vi "Read Measurement (Statistics).vi"(0 "VISA resource name":refnum<visa-resource-name>, 5 "Statistics Type (0: All)":i32(ring) items=["All", "Current", "Minimum", "Maximum", "Mean", "Std Dev", "Count"], 11 "error in (no error)":errorcluster) -> (2 "Measurement Data":string[](array[string]), 3 "Current Data":dbl[](array[numeric]), 4 "VISA resource name out":refnum<visa-resource-name>, 6 "Mean Data":dbl[](array[numeric]), 8 "Minimum Data":dbl[](array[numeric]), 10 "Maximum Data":dbl[](array[numeric]), 13 "Count Data":dbl[](array[numeric]), 14 "Std Dev Data":dbl[](array[numeric]), 15 "error out":errorcluster)   [LabVIEW 2015, in "Agilent 2000 3000 X-Series.lvlib"]
doc: "Returns the measurement of static acquisition."
uses:
  <instrlib>/Agilent 2000 3000 X-Series/Agilent 2000 3000 X-Series.lvlib
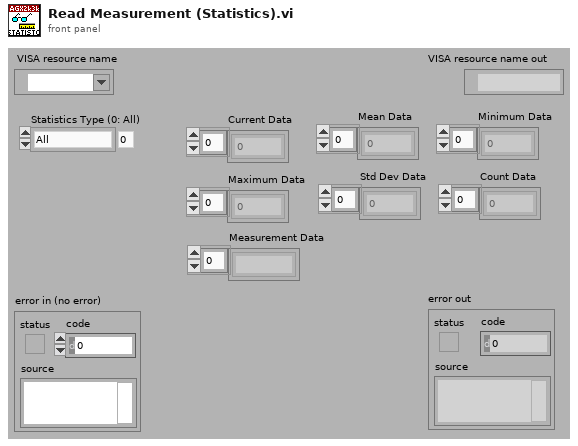
[diagram p1: front panel]
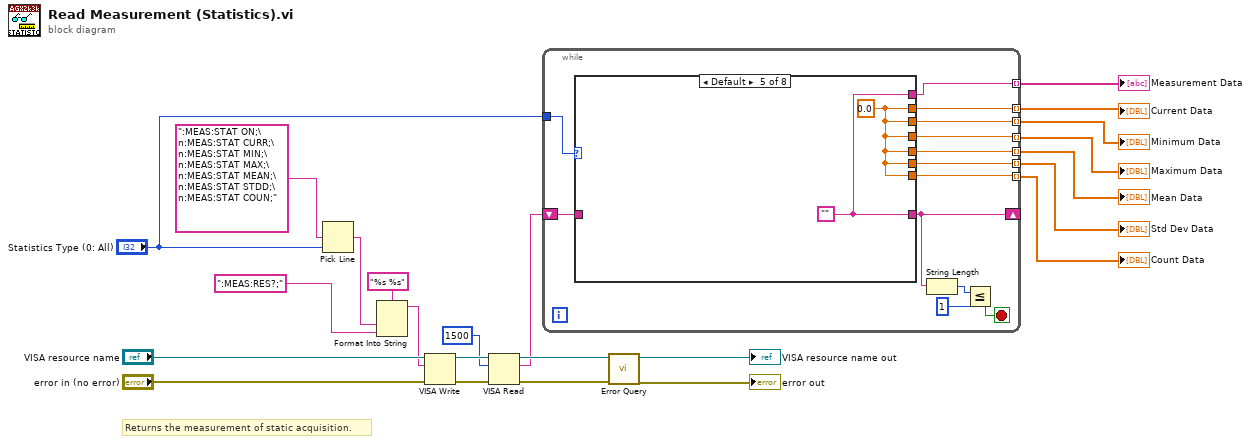
[diagram p0: block diagram]
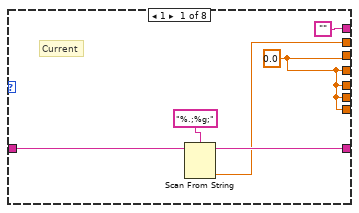
[diagram p2: hidden frame]
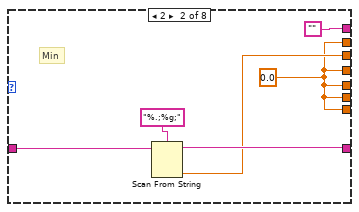
[diagram p3: hidden frame]
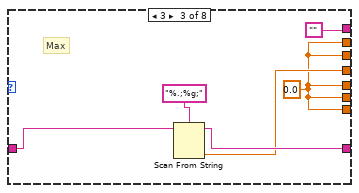
[diagram p4: hidden frame]
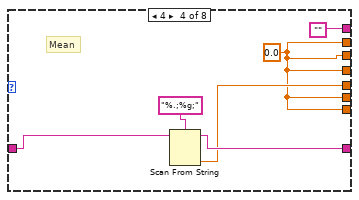
[diagram p5: hidden frame]
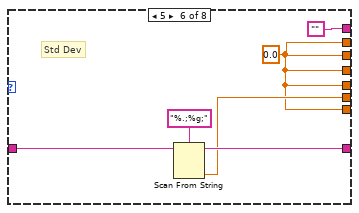
[diagram p6: hidden frame]
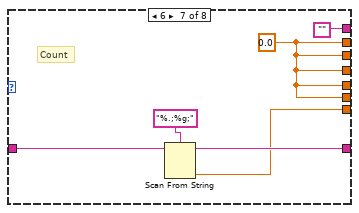
[diagram p7: hidden frame]
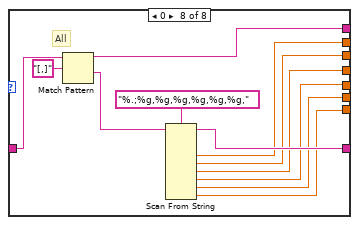
[diagram p8: hidden frame]
diagram:
  # "Returns the measurement of static acquisition."
  n1 = Pick Line(multi-line string=":MEAS:STAT ON;\n:MEAS:STAT CURR;\n:MEAS:STAT MIN;\n:MEAS:STAT MAX;\n:MEAS:STAT MEAN;\n:MEAS:STAT STDD;\n:MEAS:STAT COUN;", line index="Statistics Type (0: All)") -> (output string=w17:string)  [unwired: 1 out]
  n2 = Format Into String(format string="%s %s", w17, ":MEAS:RES?;") -> (resulting string=w15:string)  [unwired: 2 in, 1 out]
  n3 = VISA Write(VISA resource name="VISA resource name", write buffer=w15, error in (no error)="error in (no error)") -> (VISA resource name out=w14:refnum<visa-resource-name>, error out=w13:errorcluster)  [unwired: 1 out]
  n4 = VISA Read(VISA resource name=w14, byte count=u32 1500, error in (no error)=w13) -> (VISA resource name out=w12:refnum<visa-resource-name>, read buffer=w8:string, error out=w11:errorcluster)  [unwired: 1 out]
  n5 = while {
    tunnel: "Statistics Type (0: All)" -> [w36]
    shift-right: [w27] -> _
    shift-left: w8 -> [w35]
    tunnel: [w34] -> w7 mode=indexing
    tunnel: [w33] -> w6 mode=indexing
    tunnel: [w32] -> w5 mode=indexing
    tunnel: [w31] -> w4 mode=indexing
    tunnel: [w30] -> w3 mode=indexing
    tunnel: [w29] -> w2 mode=indexing
    tunnel: [w28] -> w1 mode=indexing
    stop <- w24 stop-if-true
    n6 = case shown="Default" w36 {
      tunnel: [w41 w46 w52 w58 w61 w66 w72 w85] -> w27
      tunnel: w35 -> [w40 w47 w53 w59 _ w67 w73 w76]
      tunnel: ["" "" "" "" w61 "" "" w84] -> w34
      tunnel: [w39 w44 w50 w56 w62 w64 w70 w83] -> w33
      tunnel: [w38 w45 w50 w56 w62 w64 w70 w82] -> w32
      tunnel: [w38 w44 w51 w56 w62 w64 w70 w81] -> w31
      tunnel: [w38 w44 w50 w57 w62 w64 w70 w80] -> w30
      tunnel: [w38 w44 w50 w56 w62 w65 w70 w79] -> w29
      tunnel: [w38 w44 w50 w56 w62 w64 w71 w78] -> w28
      frame 1 {
        w38 = 0.0
        # "Current"
        n7 = Scan From String(format string="%.;%g;", input string=w40) -> (remaining string=w41:string, output 1=w39:dbl)  [unwired: 2 in, 3 out]
      }
      frame 2 {
        w44 = 0.0
        # "Min"
        n8 = Scan From String(format string="%.;%g;", input string=w47) -> (remaining string=w46:string, output 1=w45:dbl)  [unwired: 2 in, 3 out]
      }
      frame 3 {
        w50 = 0.0
        # "Max"
        n9 = Scan From String(format string="%.;%g;", input string=w53) -> (remaining string=w52:string, output 1=w51:dbl)  [unwired: 2 in, 3 out]
      }
      frame 4 {
        w56 = 0.0
        # "Mean"
        n10 = Scan From String(format string="%.;%g;", input string=w59) -> (remaining string=w58:string, output 1=w57:dbl)  [unwired: 2 in, 3 out]
      }
      frame Default {
        w61 = ""
        w62 = 0.0
      }
      frame 5 {
        w64 = 0.0
        # "Std Dev"
        n11 = Scan From String(format string="%.;%g;", input string=w67) -> (remaining string=w66:string, output 1=w65:dbl)  [unwired: 2 in, 3 out]
      }
      frame 6 {
        w70 = 0.0
        # "Count"
        n12 = Scan From String(format string="%.;%g;", input string=w73) -> (remaining string=w72:string, output 1=w71:dbl)  [unwired: 2 in, 3 out]
      }
      frame 0 {
        # "All"
        n13 = Match Pattern(string=w76, regular expression="[,]") -> (before substring=w84:string, after substring=w77:string)  [unwired: 3 out]
        n14 = Scan From String(format string="%.;%g,%g,%g,%g,%g,%g,", input string=w77) -> (remaining string=w85:string, output 1=w83:dbl, output 2=w82:dbl, output 3=w81:dbl, output 4=w80:dbl, output 5=w79:dbl, output 6=w78:dbl)  [unwired: 2 in, 8 out]
      }
    }
    n15 = String Length(string=w27) -> (length=w26:i32)
    n16 = Less Or Equal?(x=w26, y=1) -> (x <= y?=w24:bool)
  }
  "Current Data" <- w6
  "Mean Data" <- w3
  "Minimum Data" <- w5
  "Maximum Data" <- w4
  "Std Dev Data" <- w2
  "Count Data" <- w1
  "Measurement Data" <- w7
  n17 = call <instrlib>:"Error Query.vi"("error in (no error)"=w11, "VISA resource name"=w12) -> ("error out"=→"error out":errorcluster, "VISA resource name out"=→"VISA resource name out":refnum<visa-resource-name>)  [unwired: 8 out]
